vi "黑盾空调.vi"() -> ()   [LabVIEW 2016, in "环境动力监测库.lvlib" / "空调库.lvlib"]
uses:
  <vilib>/Utility/config.llb/NI_LVConfig.lvlib
  <vilib>/ptbypt/NI_PtbyPt.lvlib
panel:
  in  "重开串口":bool
  in  "校时":bool
  in  "设定参数":bool
  in  "遥控":bool
  out "获取设备厂家信息":T1
  out "仪器时间":timestamp
  out "获取参数(定点数)":T2
  out "机柜空调告警状态":T3
  out "开关量输入状态解析":T4
  out "系统模拟量量化数据":T5
  out "写入缓冲区":string
  out "读取缓冲区":string
  out "source":string
  out "读取选择":string(combo)
  out "通讯":bool
  in  "VISA resource name":refnum<visa-resource-name>="COM10" caption="VISA资源名称"
  # "黑盾空调"
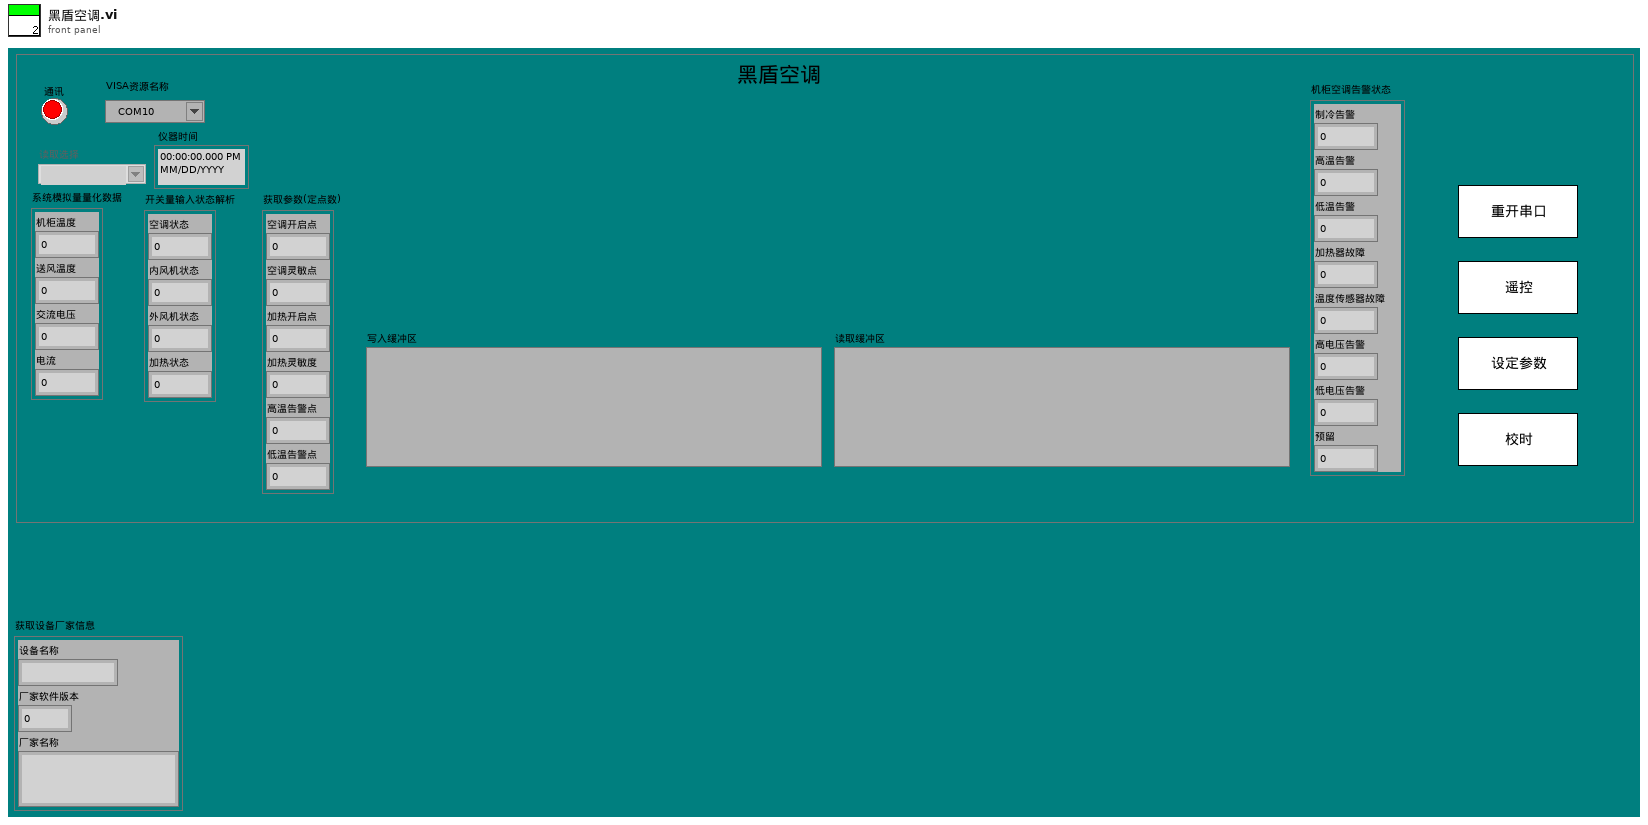
[diagram p1: front panel]
types:
  T1 = cluster{"设备名称":string, "厂家软件版本":u16, "厂家名称":string}
  T2 = cluster{"空调开启点":u16, "空调灵敏点":u16, "加热开启点":u16, "加热灵敏度":u16, "高温告警点":u16, "低温告警点":u16}
  T3 = cluster{"制冷告警":u16, "高温告警":u16, "低温告警":u16, "加热器故障":u16, "温度传感器故障":u16, "高电压告警":u16, "低电压告警":u16, "预留":u16}
  T4 = cluster{"空调状态":u16, "内风机状态":u16, "外风机状态":u16, "加热状态":u16}
  T5 = cluster{"机柜温度":sgl, "送风温度":sgl, "交流电压":sgl, "电流":sgl}
  T6 = cluster{"分支":enum16{"open", "read", "write", "close"}, "字符串":string}
  T7 = cluster{"分支":enum16{"open", "read", "write", "close"}, "读取选择":string}
  T8 = typedef "NI_LVConfig.lvlib/Config Data RefNum.ctl" = refnum<k1>
  T9 = enum16{"获取模拟量量化数据（浮点数）", "获取模拟量量化数据（定点数）", "获取开关输入状态", "获取机柜空调告警状态", "遥控", "获取系统参数（浮点数）", "获取系统参数（定点数）", "设定系统参数（浮点数）", "设定系统参数（定点数）", "获取系统历史数据（浮点数）", "获取系统历史数据（定点数）", "获取历史告警", "获取监测模块时间", "设定监测模块时间", "获取通信协议版本号", "获取设备地址", "获取设备厂家信息", "设定设备地址（ADR）"}
  T10 = cluster{"分支":enum16{"open", "read", "write", "close"}, "连接的字符串":string}
  T11 = cluster{"漏水监测输出":bool, "门禁监测输出":bool, "温湿度监测输出":bool, "烟雾监测输出":bool, "空调监测输出":bool, "自动重合闸输出":bool}
  T12 = enum16{"空调开机", "空调关机", "制冷开启", "制冷关闭", "制热开启", "制热关闭"}
  T13 = enum16{"空调开启点", "空调灵敏点", "加热开启点", "加热灵敏度", "高温告警点", "低温告警点"}
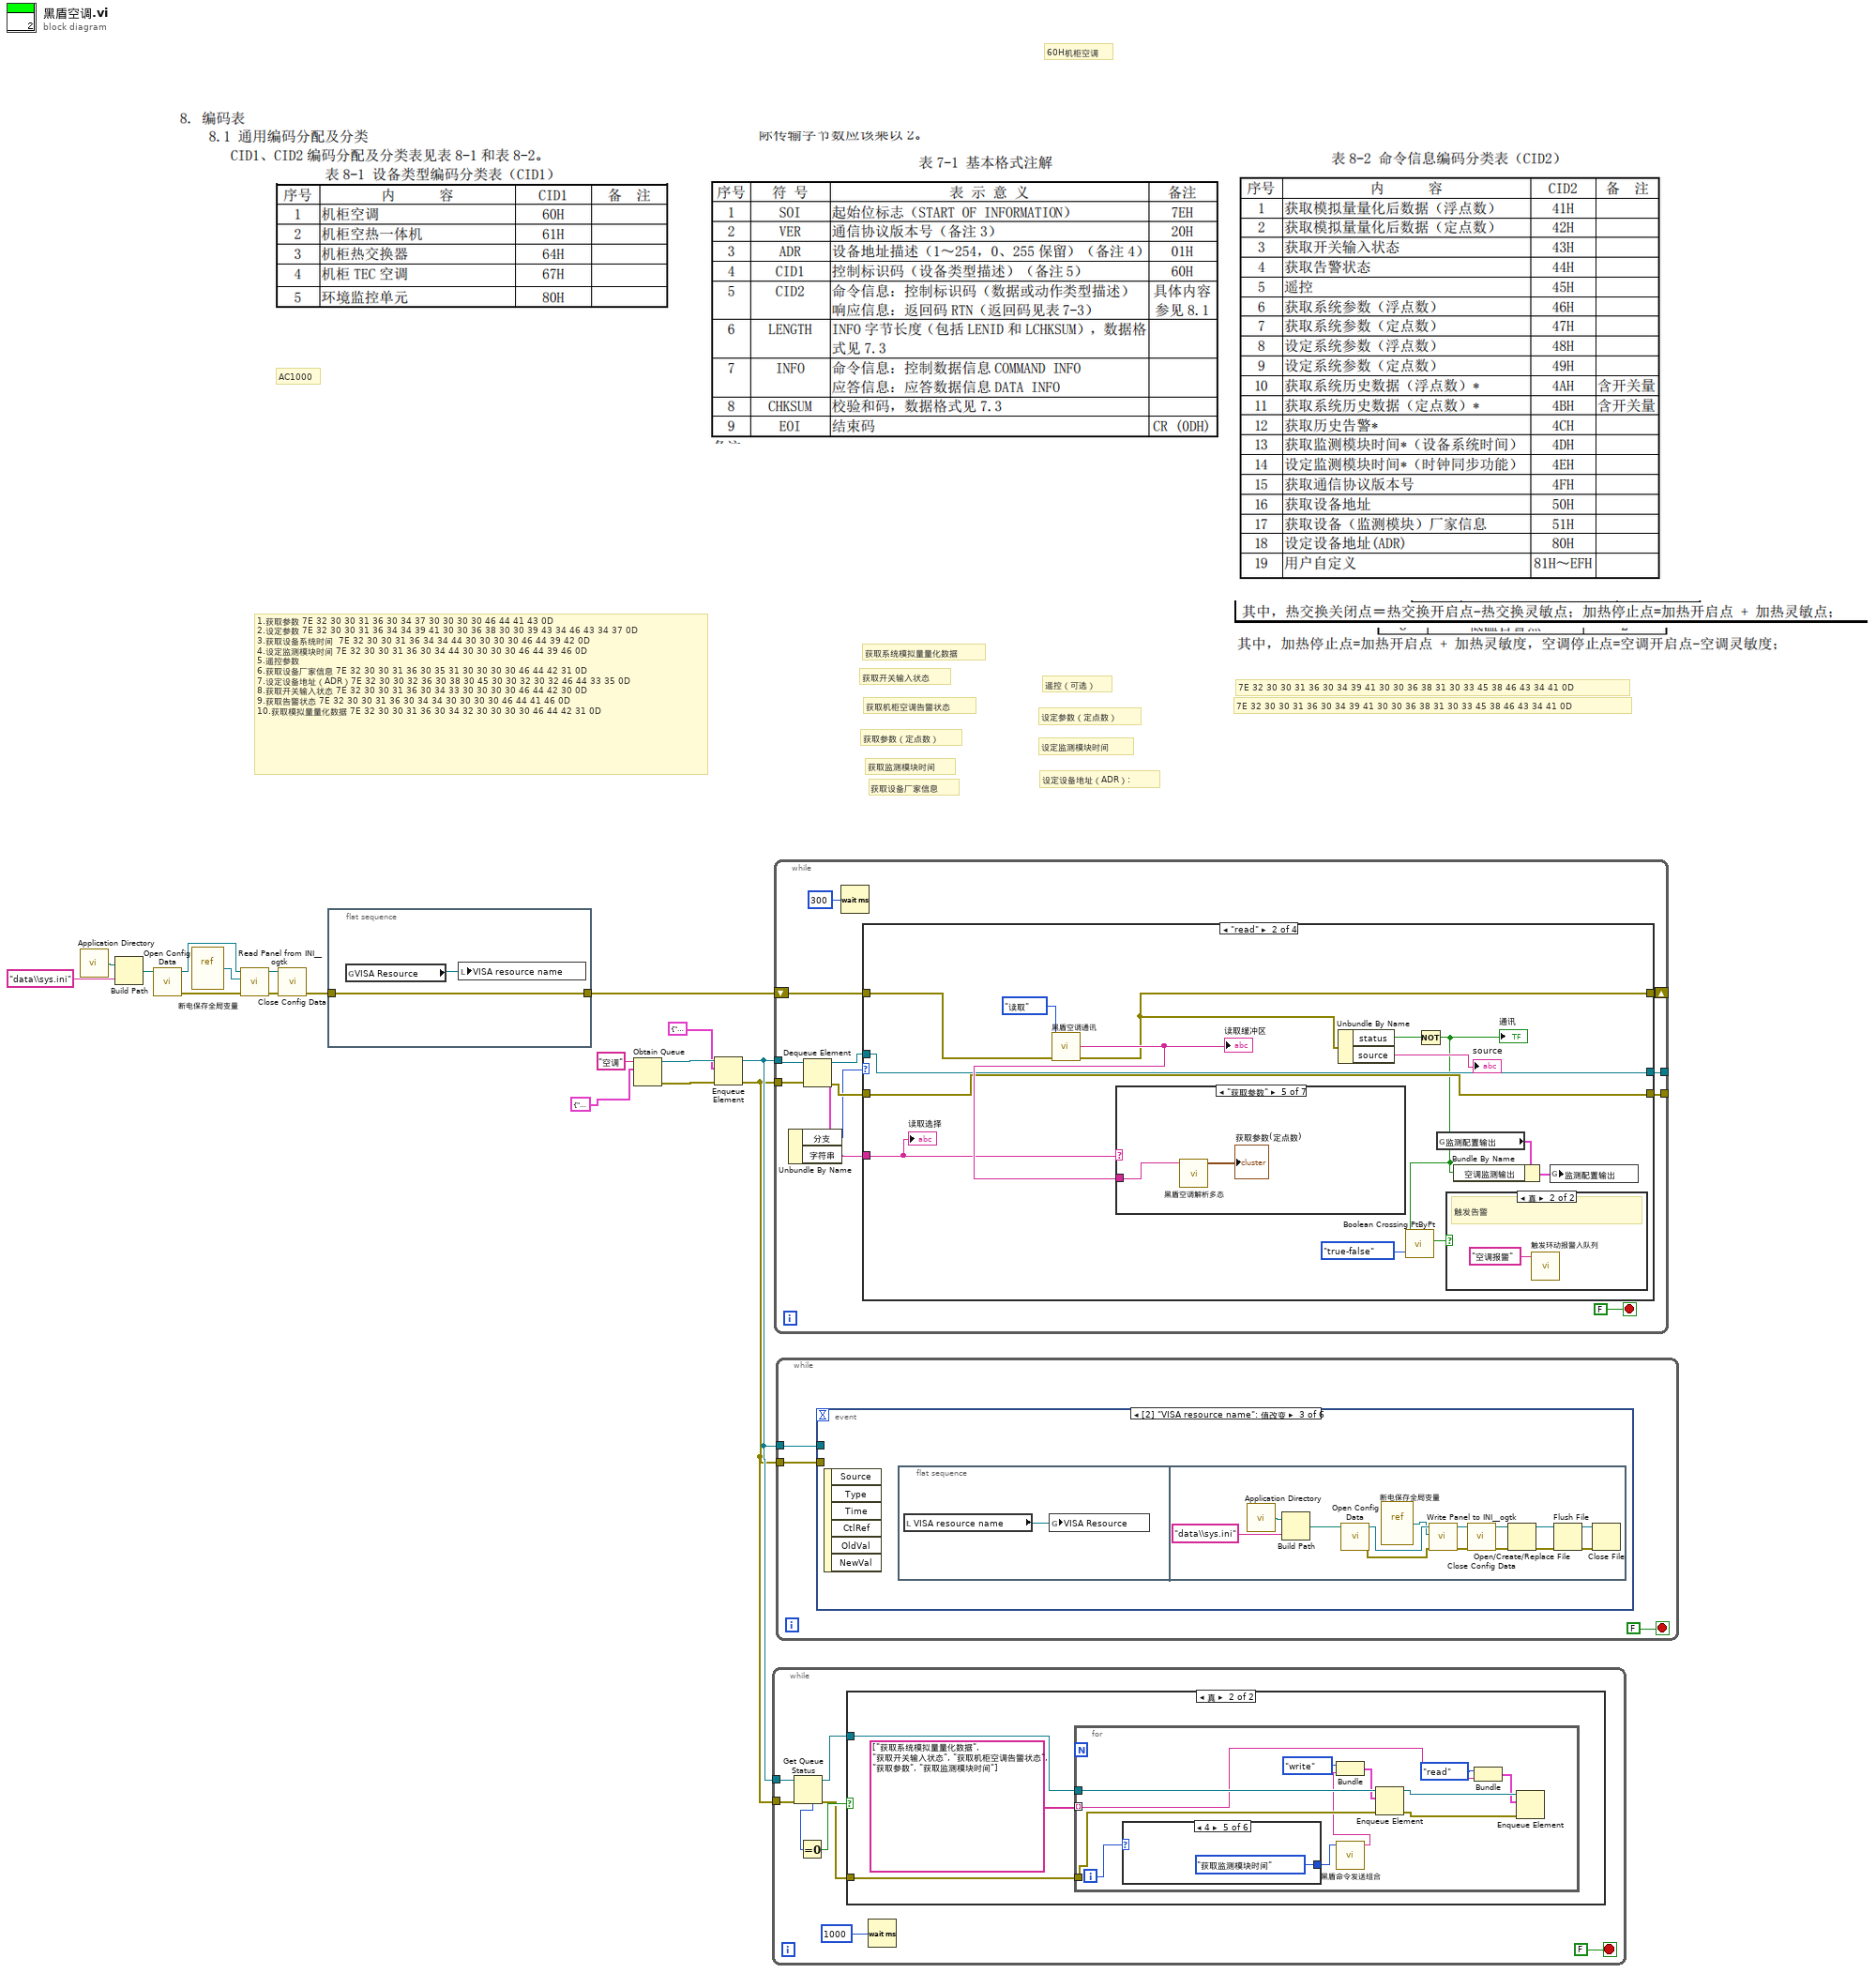
[diagram p0: block diagram]
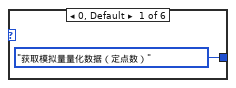
[diagram p3: hidden frame]
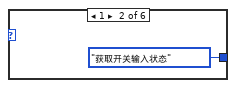
[diagram p4: hidden frame]
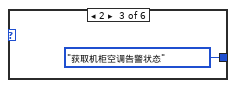
[diagram p5: hidden frame]
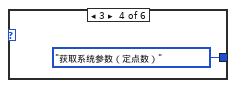
[diagram p6: hidden frame]
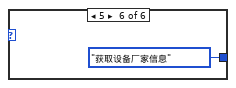
[diagram p7: hidden frame]
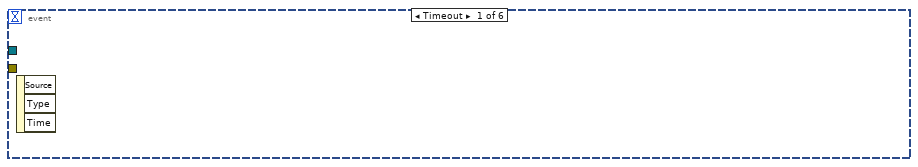
[diagram p8: hidden frame]
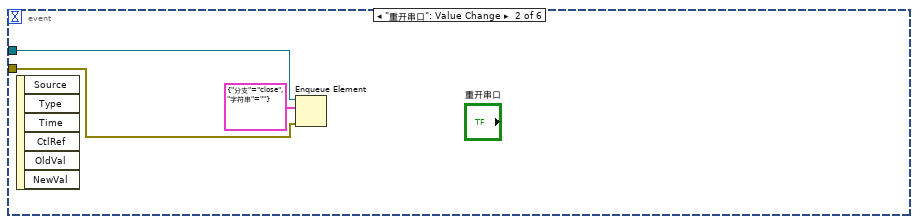
[diagram p9: hidden frame]
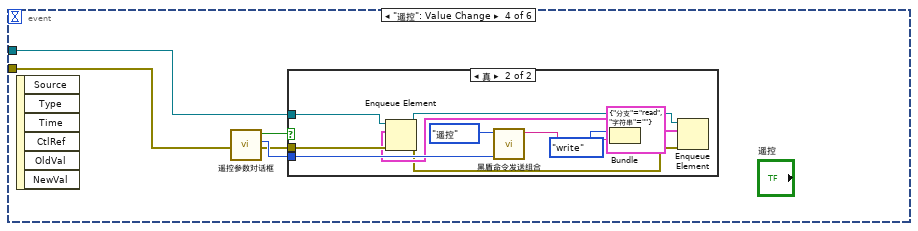
[diagram p10: hidden frame]
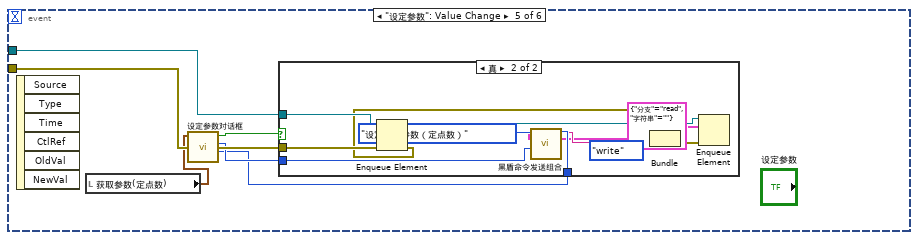
[diagram p12: hidden frame]
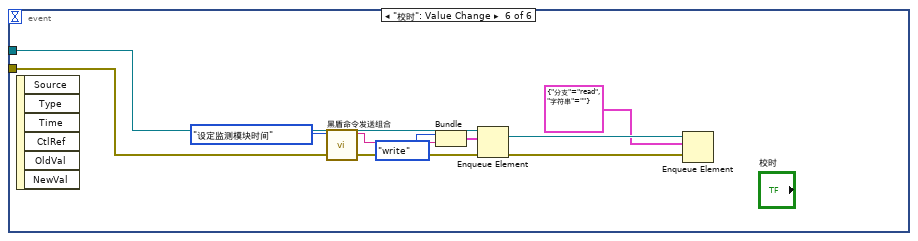
[diagram p14: hidden frame]
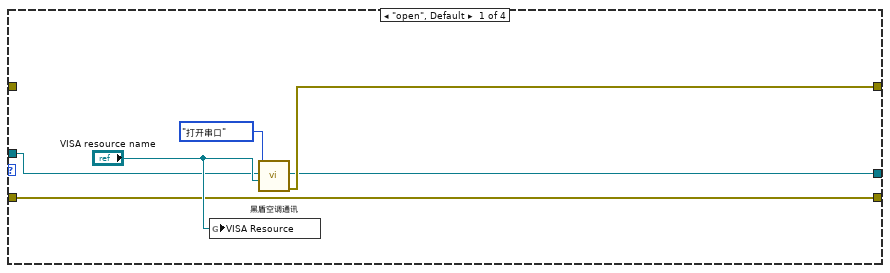
[diagram p15: hidden frame]
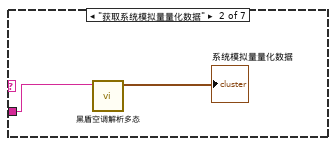
[diagram p18: hidden frame]
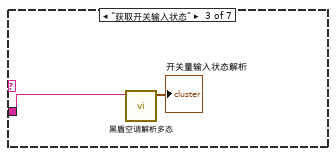
[diagram p19: hidden frame]
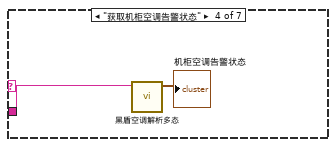
[diagram p20: hidden frame]
diagram:
  # "获取系统模拟量量化数据"
  # "设定设备地址（ADR）:"
  # "获取设备厂家信息"
  # "设定监测模块时间"
  # "获取监测模块时间"
  # "设定参数（定点数）"
  # "获取参数（定点数）"
  # "遥控（可选）"
  # "获取机柜空调告警状态"
  # "获取开关输入状态"
  # "7E 32 30 30 31 36 30 34 39 41 30 30 36 38 31 30 33 45 38 46 43 34 41 0D"
  # "7E 32 30 30 31 36 30 34 39 41 30 30 36 38 31 30 33 45 38 46 43 34 41 0D"
  # "60H机柜空调"
  # "AC1000"
  # "1.获取参数 7E 32 30 30 31 36 30 34 37 30 30 30 30 46 44 41 43 0D\n2.设定参数 7E 32 30 30 31 36 34 34 39 41 30 30 36 38 30 30 39 43 34 46 43 34 37 0D \n3.获取设备系统时间  7E 32 30 30 31 36 34 34 44 30 30 30 30 46 44 39 42 0D\n4.设定监测模块时间 7E 32 30 30 31 36 30 34 44 30 30 30 30 46 44 39 46 0D\n5.遥控参数\n6.获取设备厂家信息 7E 32 30 30 31 36 30 35 31 30 30 30 30 46 44 42 31 0D\n7.设定设备地址（ADR）7E 32 30 30 32 36 30 38 30 45 30 30 32 30 32 46 44 33 35 0D\n8.获取开关输入状态 7E 32 30 30 31 36 30 34 33 30 30 30 30 46 44 42 30 0D\n9.获取告警状态 7E 32 30 30 31 36 30 34 34 30 30 30 30 46 44 41 46 0D\n10.获取模拟量量化数据 7E 32 30 30 31 36 30 34 32 30 30 30 30 46 44 42 31 0D"
  n1 = call <vilib>:"Application Directory.vi"() -> ("Application Directory"=w17:path)
  n2 = Build Path(base path=w17, name or relative path="data\\sys.ini" ("名称或相对路径")) -> (appended path=w15:path)
  n3 = call <vilib>:"Open Config Data.vi"("configuration file path"=w15) -> ("error out"=w11:errorcluster, "refnum"=w14:T8)  [unwired: 8 in, 1 out]
  n4 = vi-ref "断电保存全局变量.vi"() -> (w13:refnum<vi>)
  n5 = call <userlib>:"Read Panel from INI__ogtk.vi"("error in (no error)"=w11, "VI ref"=w13, "refnum"=w14) -> ("error out"=w10:errorcluster, "refnum out"=w12:T8)  [unwired: 7 in]
  n6 = call <vilib>:"Close Config Data.vi"("error in (no error)"=w10, "refnum"=w12) -> ("error out"=w9:errorcluster)  [unwired: 8 in, 1 out]
  n7 = flat-sequence {
    tunnel: w9 -> [w18]
    tunnel: [w18] -> w8
    frame #0 {
      n8 = global read "断电保存全局变量.vi" "VISA Resource"() -> (w19:refnum<visa-resource-name>)
      n9 = local write "VISA resource name"(w19) -> ()
    }
  }
  n10 = Obtain Queue(name (unnamed)="空调" ("名称（未命名）"), element data type=T6 {"分支"=enum."open", "字符串"="获取系统模拟量量化数据"}) -> (queue out=w6:refnum<queue>, error out=w5:errorcluster)  [unwired: 3 in, 1 out]
  n11 = Enqueue Element(queue=w6, element=T7 {"分支"=enum."open", "读取选择"="获取系统模拟量量化数据"}, error in (no error)=w5) -> (queue out=w4:refnum<queue>, error out=w3:errorcluster)  [unwired: 1 in, 1 out]
  n12 = while {
    tunnel: w4 -> [w26]
    tunnel: w3 -> [w25]
    stop <- FALSE stop-if-true
    n13 = Get Queue Status(queue=w26, error in (no error)=w25) -> (queue out=w22:refnum<queue>, error out=w21:errorcluster, # elements in queue=w24:i32)  [unwired: 1 in, 5 out]
    n14 = Equal To 0?(x=w24) -> (x = 0?=w23:bool)
    n15 = case shown="真" w23 {
      tunnel: w22 -> [_ w29]
      tunnel: w21 -> [_ w28]
      frame False {
      }
      frame True {
        n16 = for {
          tunnel: string[] ["获取系统模拟量量化数据", "获取开关输入状态", "获取机柜空调告警状态", "获取参数", "获取监测模块时间"] -> [w32] mode=indexing
          tunnel: w29 -> [w42]
          tunnel: w28 -> [w41]
          i -> [w40]
          n17 = case shown="4" w40 {
            tunnel: [T9."获取模拟量量化数据（定点数）" ("CID2枚举") T9."获取开关输入状态" ("CID2枚举") T9."获取机柜空调告警状态" ("CID2枚举") T9."获取系统参数（定点数）" ("CID2枚举") T9."获取监测模块时间" ("CID2枚举") T9."获取设备厂家信息" ("CID2枚举")] -> w39
            frame 0, Default {
            }
            frame 1 {
            }
            frame 2 {
            }
            frame 3 {
            }
            frame 4 {
            }
            frame 5 {
            }
          }
          n18 = call "黑盾命令发送组合.vi"("CID2枚举"=w39) -> ("连接的字符串"=w37:string)  [unwired: 10 in]
          n19 = Bundle("分支"=enum16{"open", "read", "write", "close"}."write", "连接的字符串"=w37) -> (w36:T10)  [unwired: 1 in]
          n20 = Enqueue Element(queue=w42, element=w36, error in (no error)=w41) -> (queue out=w34:refnum<queue>, error out=w33:errorcluster)  [unwired: 1 in, 1 out]
          n21 = Bundle("分支"=enum16{"open", "read", "write", "close"}."read", "读取选择"=w32) -> (w31:T7)  [unwired: 1 in]
          n22 = Enqueue Element(queue=w34, element=w31, error in (no error)=w33) -> ()  [unwired: 1 in, 3 out]
        }
      }
    }
    n23 = Wait (ms)(milliseconds to wait=u32 1000 ("等待时间（毫秒）")) -> ()  [unwired: 1 out]
  }
  n24 = while {
    tunnel: w4 -> [w59]
    tunnel: w3 -> [w58]
    shift-right: [w57] -> _
    shift-left: w8 -> [w56]
    tunnel: [w53] -> _
    tunnel: [w52] -> _
    stop <- FALSE stop-if-true
    n25 = Dequeue Element(queue=w59, error in (no error)=w58) -> (queue out=w55:refnum<queue>, element=w51:T6, error out=w54:errorcluster)  [unwired: 1 in, 1 out]
    n26 = Unbundle By Name(w51) -> ("分支"=w50:enum16{"open", "read", "write", "close"}, "字符串"=w49:string)
    n27 = Wait (ms)(milliseconds to wait=u32 300 ("等待时间（毫秒）")) -> ()  [unwired: 1 out]
    n28 = case shown="\"read\"" w50 {
      tunnel: [w64 w72 w97 w105] -> w57
      tunnel: w56 -> [_ w79 w98 w106]
      tunnel: w55 -> [w63 w77 w95 w104]
      tunnel: w54 -> [w62 w76 w94 w103]
      tunnel: [w63 w77 w95 w101] -> w53
      tunnel: [w62 w76 w94 w100] -> w52
      tunnel: w49 -> [_ w74 w96 _]
      frame "open", Default {
        n29 = global write "断电保存全局变量.vi" "VISA Resource"("VISA resource name") -> ()
        n30 = call "黑盾空调通讯.vi"("VISA resource name"="VISA resource name", "功能输入"=enum16{"打开串口", "写入", "读取", "关闭串口"}."打开串口") -> ("error out"=w64:errorcluster)  [unwired: 7 in, 2 out]
      }
      frame "read" {
        n31 = call "黑盾空调通讯.vi"("error in (no error)"=w79, "功能输入"=enum16{"打开串口", "写入", "读取", "关闭串口"}."读取") -> ("error out"=w72:errorcluster, "读取缓冲区"=w78:string)  [unwired: 7 in, 1 out]
        "读取缓冲区" <- w78
        n32 = case shown="\"获取参数\"" w74 {
          tunnel: w78 -> [_ w83 w85 w87 w89 w91 w93]
          frame "假", Default {
          }
          frame "获取系统模拟量量化数据" {
            n33 = call-poly "黑盾空调解析多态.vi"("输入字符串"=w83) -> ("系统模拟量量化数据"=→"系统模拟量量化数据":T5)  [unwired: 10 in]
          }
          frame "获取开关输入状态" {
            n34 = call-poly "黑盾空调解析多态.vi"("输入字符串"=w85) -> ("开关量输入状态解析"=→"开关量输入状态解析":T4)  [unwired: 10 in]
          }
          frame "获取机柜空调告警状态" {
            n35 = call-poly "黑盾空调解析多态.vi"("输入字符串"=w87) -> ("机柜空调告警状态"=→"机柜空调告警状态":T3)  [unwired: 10 in]
          }
          frame "获取参数" {
            n36 = call-poly "黑盾空调解析多态.vi"("输入字符串"=w89) -> ("获取参数(定点数)"=→"获取参数(定点数)":T2)  [unwired: 10 in]
          }
          frame "获取监测模块时间" {
            n37 = call-poly "黑盾空调解析多态.vi"("输入字符串"=w91) -> ("时间标识"=→"仪器时间":timestamp)  [unwired: 10 in]
          }
          frame "获取设备厂家信息" {
            n38 = call-poly "黑盾空调解析多态.vi"("输入字符串"=w93) -> ("获取设备厂家信息"=→"获取设备厂家信息":T1)  [unwired: 10 in]
          }
        }
        n39 = Unbundle By Name(w72) -> ("status"=w73:bool, "source"=→"source":string)
        n40 = Not(x=w73) -> (.not. x?=w67:bool)
        "通讯" <- w67
        n41 = call <vilib>:"Boolean Crossing PtByPt.vi"("direction"=enum16{"either", "false-true", "true-false"}."true-false", "input"=w67) -> ("crossing"=w68:bool)  [unwired: 1 in]
        n42 = global read "内部交互全局变量.vi" "监测配置输出"() -> (w71:T11)
        n43 = case shown="真" w68 {
          frame False {
          }
          frame True {
            # "触发告警"
            n44 = call "触发环动报警入队列.vi"("报警内容"="空调报警") -> ()  [unwired: 11 in]
          }
        }
        n45 = Bundle By Name(cluster=w71, "空调监测输出"=w67) -> (w70:T11)
        n46 = global write "内部交互全局变量.vi" "监测配置输出"(w70) -> ()
        "读取选择" <- w74
      }
      frame "write" {
        n47 = call "黑盾空调通讯.vi"("error in (no error)"=w98, "写入缓冲区"=w96, "功能输入"=enum16{"打开串口", "写入", "读取", "关闭串口"}."写入") -> ("error out"=w97:errorcluster)  [unwired: 6 in, 2 out]
        "写入缓冲区" <- w96
      }
      frame "close" {
        n48 = call "黑盾空调通讯.vi"("error in (no error)"=w106, "功能输入"=enum16{"打开串口", "写入", "读取", "关闭串口"}."关闭串口") -> ("error out"=w105:errorcluster)  [unwired: 7 in, 2 out]
        n49 = Enqueue Element(queue=w104, element=T6 {"分支"=enum."open", "字符串"=""} ("元素"), error in (no error)=w103) -> (queue out=w101:refnum<queue>, error out=w100:errorcluster)  [unwired: 1 in, 1 out]
      }
    }
  }
  n50 = while {
    tunnel: w4 -> [w109]
    tunnel: w3 -> [w108]
    stop <- FALSE stop-if-true
    n51 = event shown="[2] \"VISA resource name\": 值改变" {
      selector: _ -> [_ _ _ _ _ _]
      dyn-events: _ -> [_ _ _ _ _ _]
      timeout: _ -> [_ _ _ _ _ _]
      tunnel: w109 -> [_ w112 _ w129 w148 w168]
      tunnel: w108 -> [_ w111 _ w130 w147 w167]
      event Timeout {
        n52 = event-data() -> ()  [unwired: 1 in, 3 out]
      }
      event "重开串口": Value Change {
        n53 = event-data() -> ()  [unwired: 1 in, 6 out]
        n54 = Enqueue Element(queue=w112, element=T6 {"分支"=enum."close", "字符串"=""} ("元素"), error in (no error)=w111) -> ()  [unwired: 1 in, 3 out]
      }
      event "VISA resource name": Value Change {
        n55 = event-data() -> ()  [unwired: 1 in, 6 out]
        n56 = flat-sequence {
          frame #0 {
            n57 = local read "VISA resource name"() -> (w114:refnum<visa-resource-name>)
            n58 = global write "断电保存全局变量.vi" "VISA Resource"(w114) -> ()
          }
          frame #1 {
            n59 = call <vilib>:"Application Directory.vi"() -> ("Application Directory"=w127:path)
            n60 = Build Path(base path=w127, name or relative path="data\\sys.ini" ("名称或相对路径")) -> (appended path=w126:path)
            n61 = call <vilib>:"Open Config Data.vi"("configuration file path"=w126) -> ("error out"=w122:errorcluster, "refnum"=w125:T8)  [unwired: 8 in, 1 out]
            n62 = vi-ref "断电保存全局变量.vi"() -> (w124:refnum<vi>)
            n63 = call <userlib>:"Write Panel to INI__ogtk.vi"("error in (no error)"=w122, "VI ref"=w124, "refnum"=w125) -> ("error out"=w121:errorcluster, "refnum out"=w123:T8)  [unwired: 7 in]
            n64 = call <vilib>:"Close Config Data.vi"("error in (no error)"=w121, "refnum"=w123) -> ("error out"=w116:errorcluster, "file path"=w115:path)  [unwired: 8 in]
            n65 = Open/Create/Replace File(file path (use dialog)=w115, error in=w116) -> (refnum out=w119:refnum<file>, error out=w120:errorcluster)  [unwired: 4 in, 1 out]
            n66 = Flush File(refnum=w119, error in=w120) -> (refnum out=w118:refnum<file>, error out=w117:errorcluster)
            n67 = Close File(refnum=w118, error in=w117) -> ()  [unwired: 2 out]
          }
        }
      }
      event "遥控": Value Change {
        n68 = event-data() -> ()  [unwired: 1 in, 6 out]
        n69 = call "遥控参数对话框.vi"() -> ("遥控参数选择输出"=w131:T12, "确定?"=w132:bool)  [unwired: 10 in]
        n70 = case shown="真" w132 {
          tunnel: w131 -> [_ w141]
          tunnel: w130 -> [_ w140]
          tunnel: w129 -> [_ w139]
          frame False {
          }
          frame True {
            n71 = call "黑盾命令发送组合.vi"("遥控参数选择"=w141, "CID2枚举"=T9."遥控") -> ("连接的字符串"=w137:string)  [unwired: 9 in]
            n72 = Bundle("分支"=enum16{"open", "read", "write", "close"}."write", "连接的字符串"=w137) -> (w136:T10)  [unwired: 1 in]
            n73 = Enqueue Element(queue=w139, element=w136, error in (no error)=w140) -> (queue out=w135:refnum<queue>, error out=w134:errorcluster)  [unwired: 1 in, 1 out]
            n74 = Enqueue Element(queue=w135, element=T6 {"分支"=enum."read", "字符串"=""} ("元素"), error in (no error)=w134) -> ()  [unwired: 1 in, 3 out]
          }
        }
      }
      event "设定参数": Value Change {
        n75 = event-data() -> ()  [unwired: 1 in, 6 out]
        n76 = local read "获取参数(定点数)"() -> (w143:T2)
        n77 = call "设定参数对话框.vi"("获取参数(定点数)"=w143) -> ("参数 2"=w144:u16, "设定参数（定点数）选择 2"=w145:T13, "确定?"=w146:bool)  [unwired: 8 in]
        n78 = case shown="真" w146 {
          tunnel: w147 -> [_ w158]
          tunnel: w148 -> [_ w157]
          tunnel: w145 -> [_ w156]
          tunnel: w144 -> [_ w155]
          frame False {
          }
          frame True {
            n79 = call "黑盾命令发送组合.vi"("参数"=w155, "设定参数（定点数）选择"=w156, "CID2枚举"=T9."设定系统参数（定点数）") -> ("连接的字符串"=w153:string)  [unwired: 8 in]
            n80 = Bundle("分支"=enum16{"open", "read", "write", "close"}."write", "连接的字符串"=w153) -> (w152:T10)  [unwired: 1 in]
            n81 = Enqueue Element(queue=w157, element=w152, error in (no error)=w158) -> (queue out=w151:refnum<queue>, error out=w150:errorcluster)  [unwired: 1 in, 1 out]
            n82 = Enqueue Element(queue=w151, element=T6 {"分支"=enum."read", "字符串"=""} ("元素"), error in (no error)=w150) -> ()  [unwired: 1 in, 3 out]
          }
        }
      }
      event "校时": Value Change {
        n83 = event-data() -> ()  [unwired: 1 in, 6 out]
        n84 = call "黑盾命令发送组合.vi"("CID2枚举"=T9."设定监测模块时间") -> ("连接的字符串"=w164:string)  [unwired: 10 in]
        n85 = Bundle("分支"=enum16{"open", "read", "write", "close"}."write", "连接的字符串"=w164) -> (w163:T10)  [unwired: 1 in]
        n86 = Enqueue Element(queue=w168, element=w163, error in (no error)=w167) -> (queue out=w162:refnum<queue>, error out=w161:errorcluster)  [unwired: 1 in, 1 out]
        n87 = Enqueue Element(queue=w162, element=T6 {"分支"=enum."read", "字符串"=""} ("元素"), error in (no error)=w161) -> ()  [unwired: 1 in, 3 out]
      }
    }
  }
